vi "DevicesManager.vi"(8 "error in (no error)":errorcluster, 10 "Notifiers":T2, 11 "All Message Queue Cluster":T3) -> (0 "error out":errorcluster)   [LabVIEW 2013]
doc: "Ce VI a pour but de géré la connection des différents appareils.\n- Il permet de les connecté en fonction de leur port.\n- Il indique s'il se sont bien connecter et si tout se passe bien."
uses:
  Lib QMH/AllMessageQueue Cluster.ctl
  Lib QMH/Message Cluster.ctl
  Lib Notifier/Notifier.ctl
  Manager UI Data.ctl
  Lib QMH/MessageQueues.lvlib
  Lib Notifier/Notifier.lvlib
panel:
  in  "Port Number Slit":T1(ring)=enum."COM3"
  out "Camera Initialized":bool
  out "Laser Initialized":bool
  out "Status Camera":string
  out "Status Laser":string
  in  "Connect Laser":bool
  in  "Connect Camera":bool
  # "Camera"
  # "Laser"
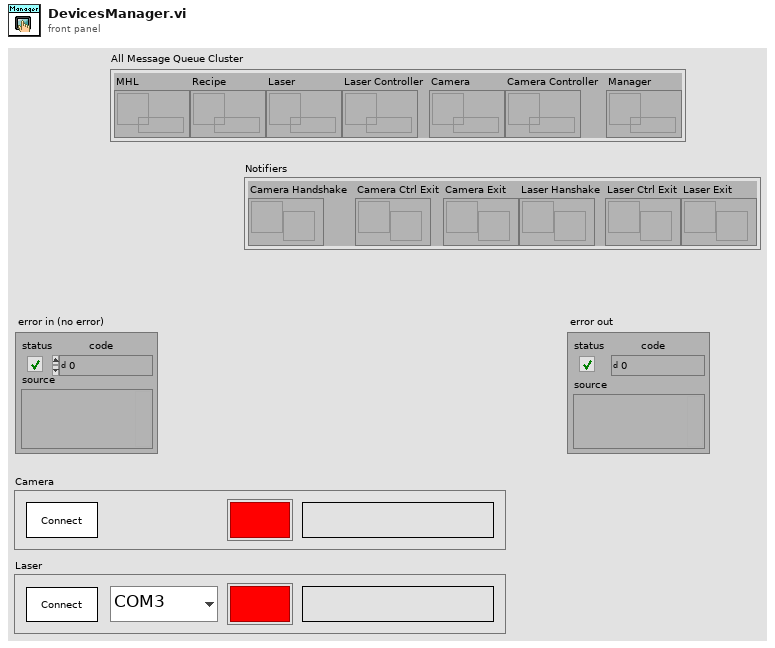
[diagram p1: front panel]
types:
  T1 = enum16{"COM1", "COM2", "COM3", "COM4", "COM5", "COM6", "COM7", "COM8", "COM9", "COM10", "COM11", "COM12", "COM13", "COM14", "COM15", "COM16", "COM17", "COM18", "COM19", "COM20", "COM21", "COM22", "COM23", "COM24", "COM25", "COM26", "COM27", "COM28", "COM29", "COM30"}
  T2 = typedef "Notifier.lvlib/Notifier.ctl" = cluster{"Camera Handshake":refnum<notifier>, "Camera Ctrl Exit":refnum<notifier>, "Camera Exit":refnum<notifier>, "Laser Hanshake":refnum<notifier>, "Laser Ctrl Exit":refnum<notifier>, "Laser Exit":refnum<notifier>}
  T3 = typedef "MessageQueues.lvlib/AllMessageQueue Cluster.ctl" = cluster{"MHL":refnum<queue>, "Recipe":refnum<queue>, "Laser":refnum<queue>, "Laser Controller":refnum<queue>, "Camera":refnum<queue>, "Camera Controller":refnum<queue>, "Manager":refnum<queue>}
  T4 = typedef "Manager UI Data.ctl" = cluster{"Camera Initialized":bool, "Status Camera":string, "Laser Initialized":bool, "Status Laser":string}
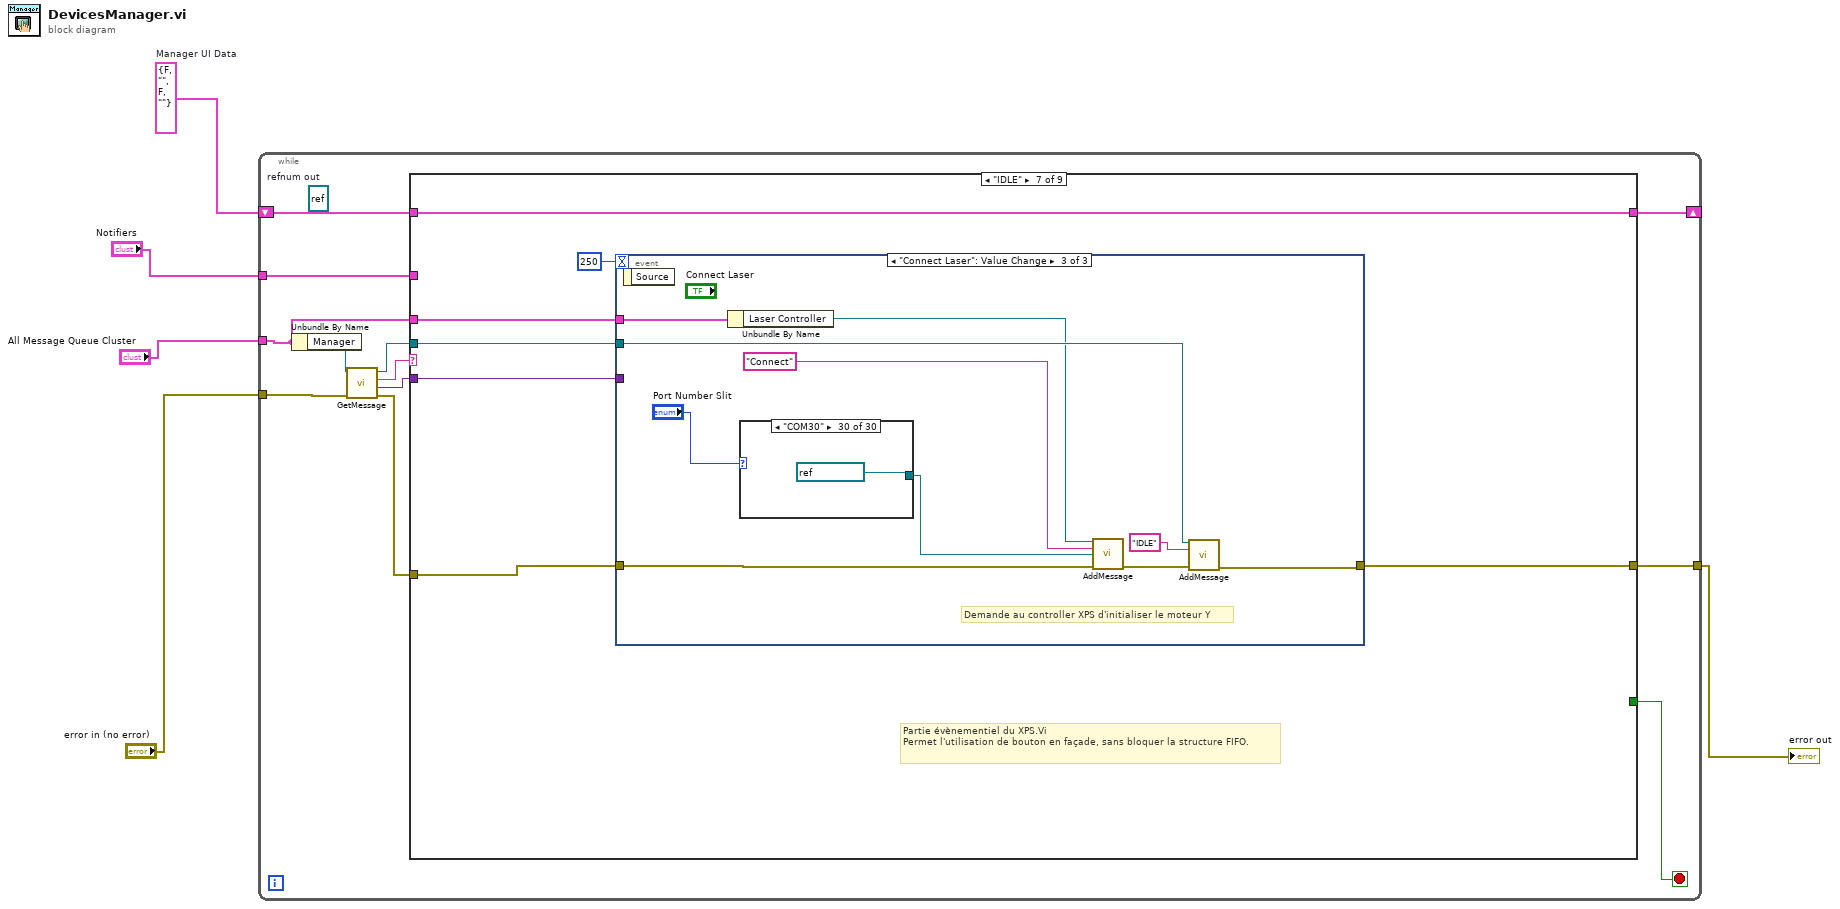
[diagram p0: block diagram]
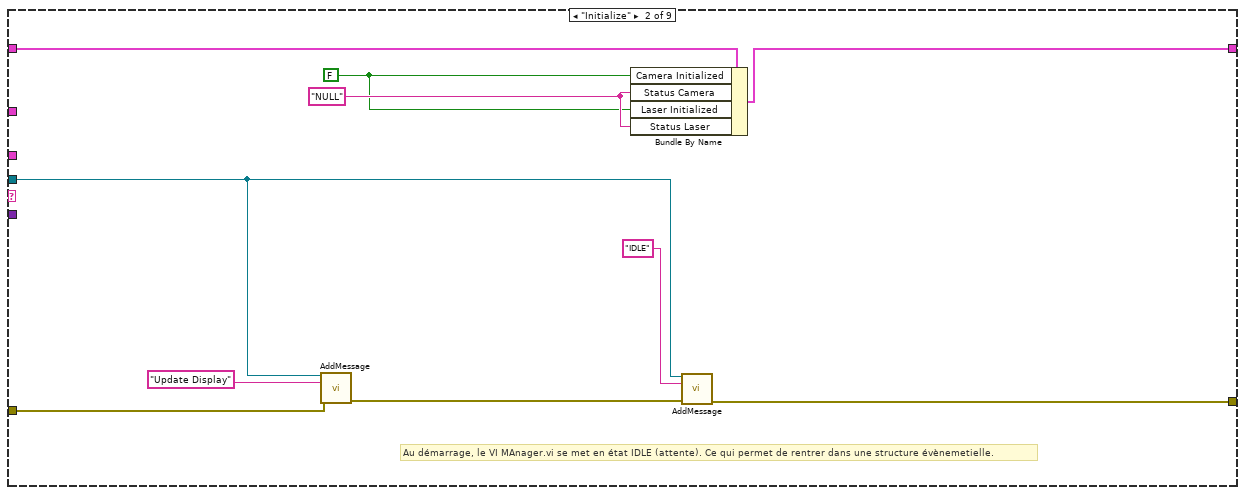
[diagram p3: hidden frame]
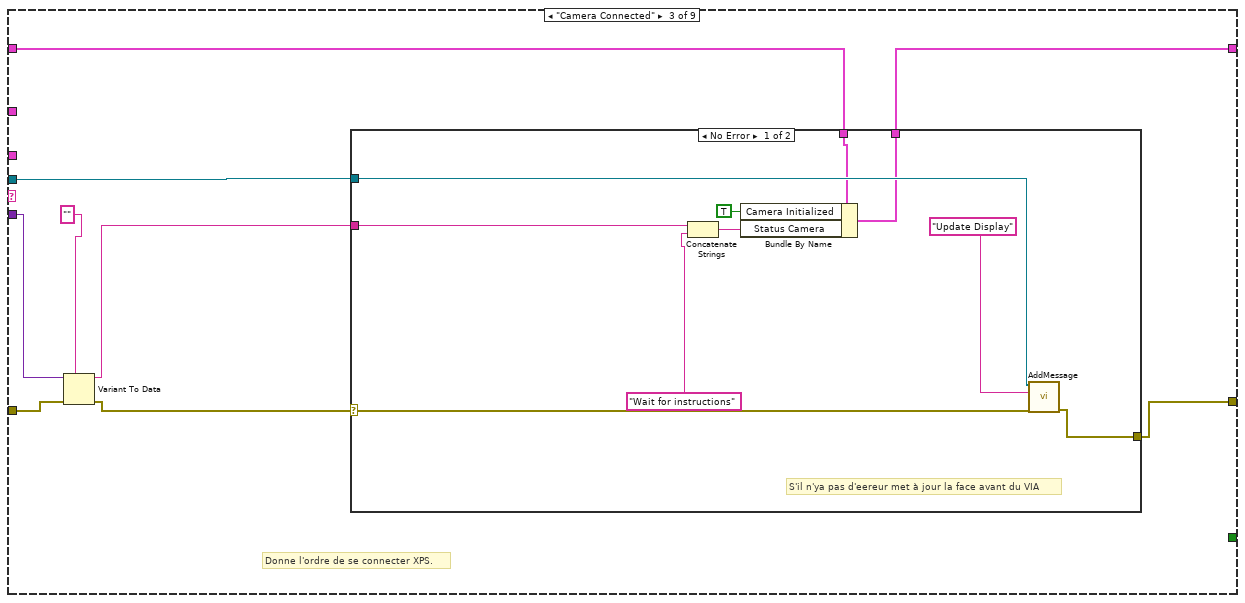
[diagram p4: hidden frame]
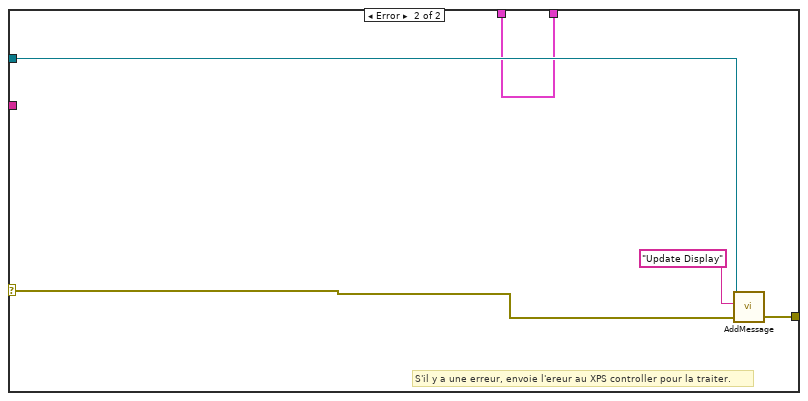
[diagram p5: hidden frame]
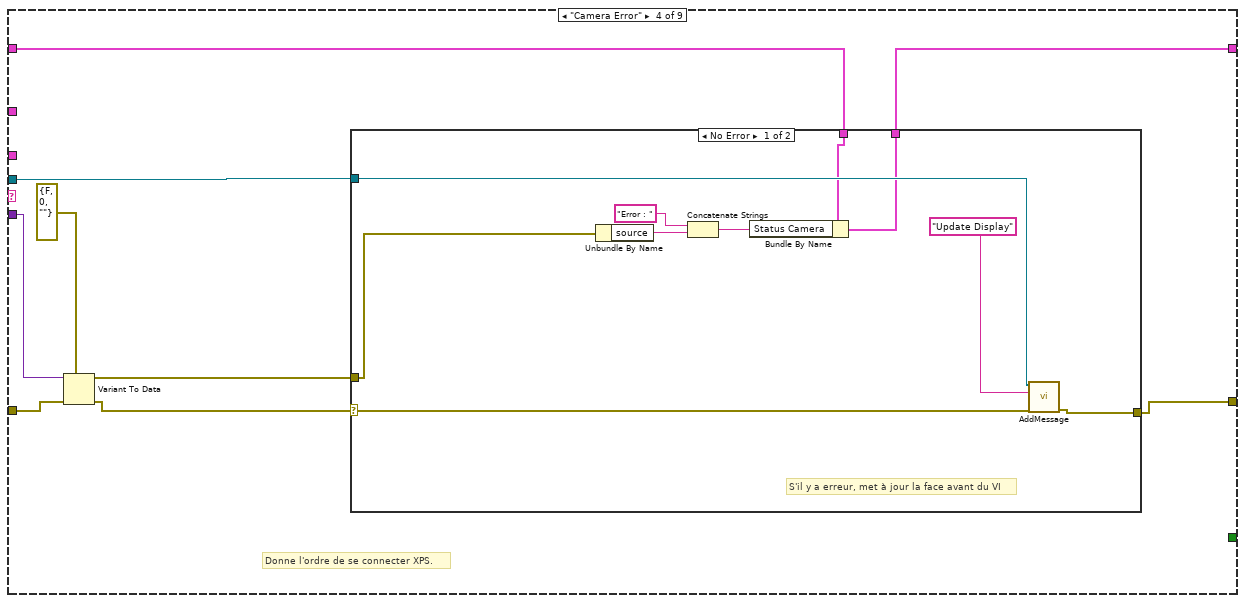
[diagram p6: hidden frame]
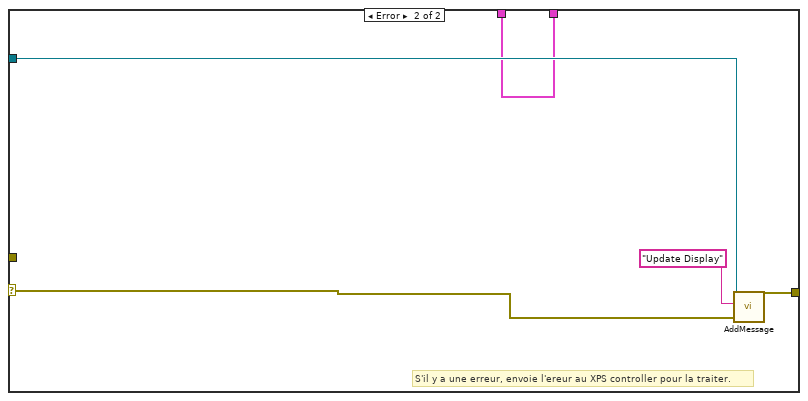
[diagram p7: hidden frame]
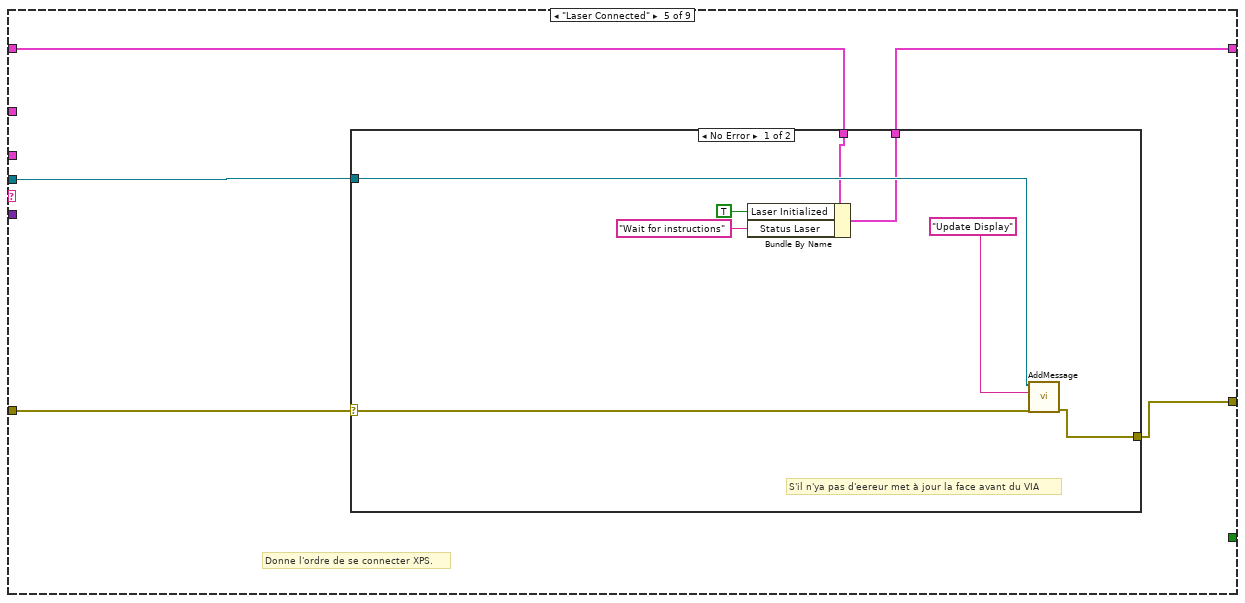
[diagram p8: hidden frame]
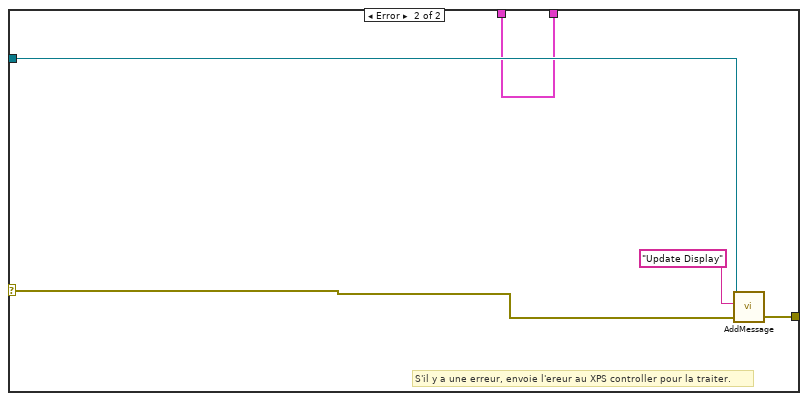
[diagram p9: hidden frame]
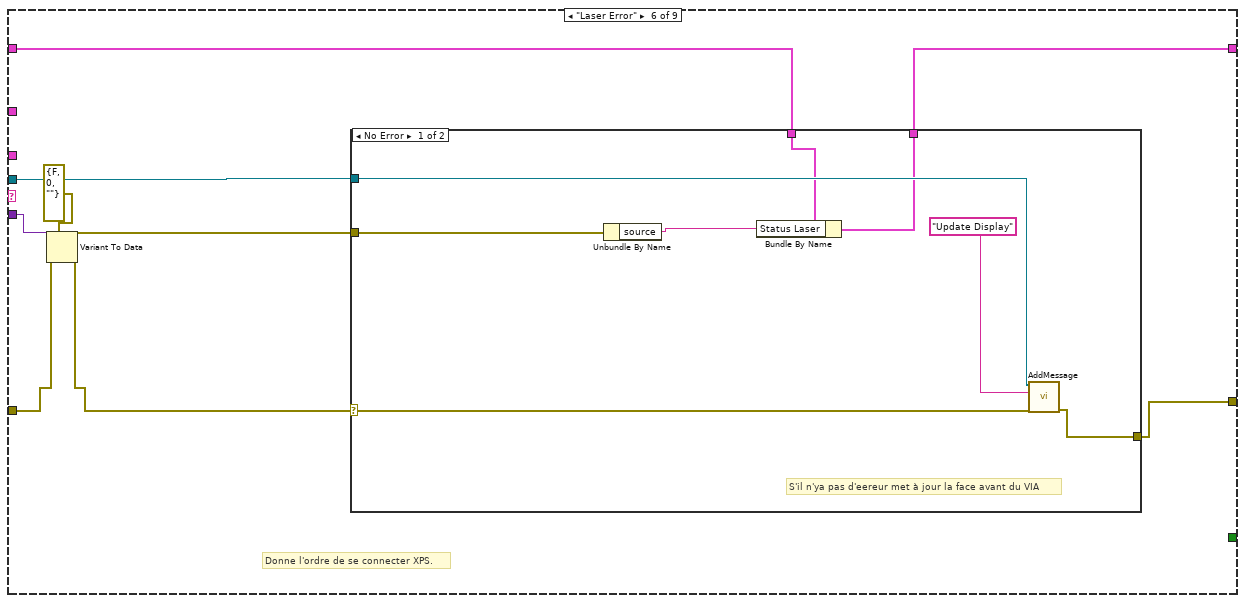
[diagram p10: hidden frame]
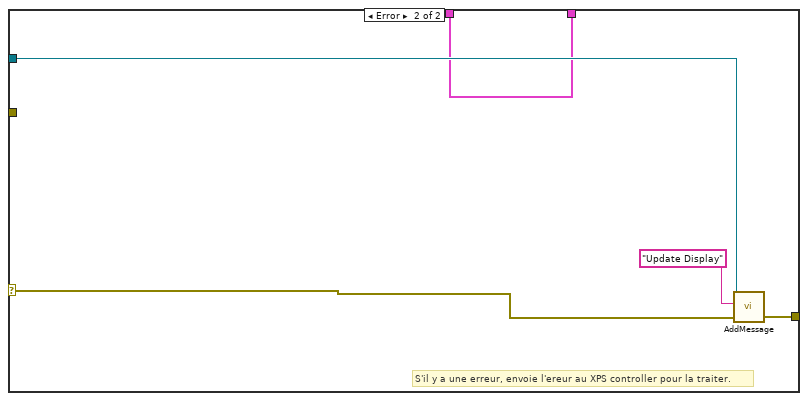
[diagram p11: hidden frame]
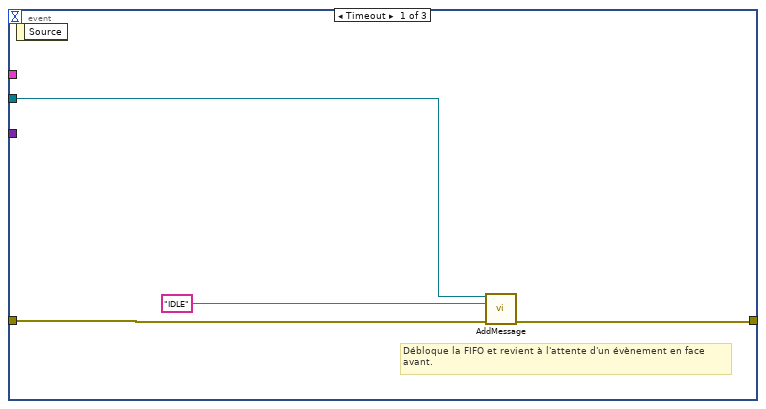
[diagram p12: hidden frame]
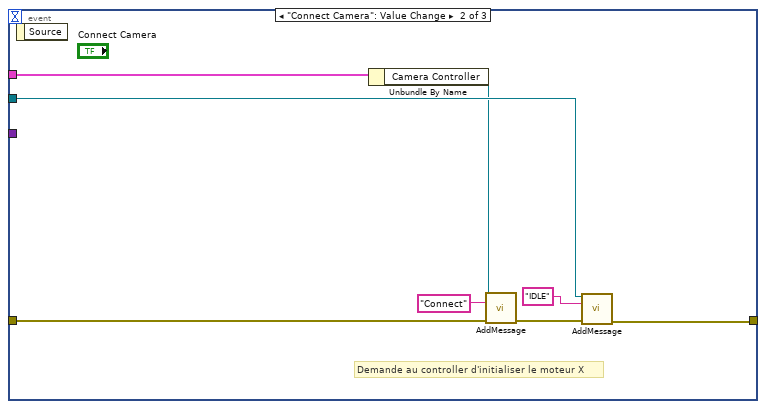
[diagram p13: hidden frame]
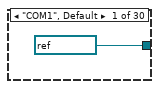
[diagram p14: hidden frame]
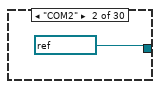
[diagram p15: hidden frame]
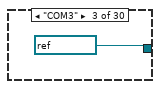
[diagram p16: hidden frame]
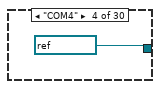
[diagram p17: hidden frame]
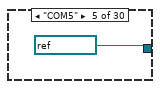
[diagram p18: hidden frame]
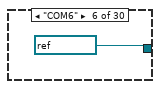
[diagram p19: hidden frame]
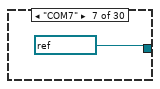
[diagram p20: hidden frame]
diagram:
  w1 = T4 {"Camera Initialized"=FALSE, "Status Camera"="", "Laser Initialized"=FALSE, "Status Laser"=""}  # Manager UI Data
  (unwired) refnum<file> refnum  # refnum out
  n1 = while {
    tunnel: "All Message Queue Cluster" -> [w6]
    tunnel: "Notifiers" -> [w17]
    tunnel: "error in (no error)" -> [w11]
    tunnel: [w10] -> w2
    shift-right: [w7] -> _
    shift-left: w1 -> [w8]
    stop <- w9 stop-if-true
    n2 = Unbundle By Name(w6) -> ("Manager"=w16:refnum<queue>)
    n3 = call "GetMessage.vi"("entrée d'erreur"=w11, "Message queue"=w16) -> ("sortie d'erreur"=w12:errorcluster, "Data"=w13:variant, "Message"=w14:string, "Dup Message Queue"=w15:refnum<queue>)  [unwired: 6 in]
    n4 = case shown="\"IDLE\"" w14 {
      tunnel: w17 -> [_ _ _ _ _ _ _ _ _]
      tunnel: w15 -> [_ w21 w38 w62 w82 w104 w123 _ w185]
      tunnel: w13 -> [_ _ w32 w56 _ w98 w122 _ _]
      tunnel: w12 -> [w19 w23 w34 w58 w78 w100 w121 w182 w186]
      tunnel: [w19 w28 w37 w61 w81 w103 w120 w182 w183] -> w10
      tunnel: [_ _ _ _ _ _ _ _ TRUE] -> w9
      tunnel: w8 -> [w18 w27 w36 w60 w80 w102 w119 w181 w184]
      tunnel: [w18 w26 w35 w59 w79 w101 w119 w181 w184] -> w7
      tunnel: w6 -> [_ _ _ _ _ _ w118 _ _]
      frame Default {
        # "ne fait rien si le message dépilé n'existe pas"
      }
      frame "Initialize" {
        w25 = "NULL" ("Status Spectro")
        w24 = FALSE ("Spectro Initialized")
        # "Au démarrage, le VI MAnager.vi se met en état IDLE (attente). Ce qui permet de rentrer dans une structure évènemetielle."
        n5 = call "AddMessage.vi"("Message queue"=w21, "Message"="Update Display", "entrée d'erreur (pas d'erreur)"=w23) -> ("error out"=w22:errorcluster)  [unwired: 11 in, 1 out]
        n6 = Bundle By Name(cluster=w27, "Camera Initialized"=w24, "Status Camera"=w25, "Laser Initialized"=w24, "Status Laser"=w25) -> (w26:T4)
        n7 = call "AddMessage.vi"("Message queue"=w21, "Message"="IDLE", "entrée d'erreur (pas d'erreur)"=w22) -> ("error out"=w28:errorcluster)  [unwired: 11 in, 1 out]
      }
      frame "Camera Connected" {
        # "Donne l'ordre de se connecter XPS."
        n8 = Variant To Data(error in=w34, type="", Variant=w32) -> (data=w30:string, error out=w33:errorcluster)
        n9 = case shown="No Error" w33 {
          selector: w33 -> [w46 w49]
          tunnel: w38 -> [w48 w53]
          tunnel: [w45 w51] -> w37
          tunnel: w36 -> [w44 w50]
          tunnel: [w43 w50] -> w35
          tunnel: w30 -> [w39 _]
          frame No Error {
            # "S'il n'ya pas d'eereur met à jour la face avant du VIA"
            n10 = Concatenate Strings(w39, "Wait for instructions" ("Status Spectro")) -> (w40:string)
            n11 = Bundle By Name(cluster=w44, "Camera Initialized"=TRUE ("Spectro Initialized"), "Status Camera"=w40) -> (w43:T4)
            n12 = call "AddMessage.vi"("Message queue"=w48, "Message"="Update Display", "entrée d'erreur (pas d'erreur)"=w46) -> ("error out"=w45:errorcluster)  [unwired: 11 in, 1 out]
          }
          frame Error {
            # "S'il y a une erreur, envoie l'ereur au XPS controller pour la traiter."
            n13 = call "AddMessage.vi"("Message queue"=w53, "Message"="Update Display", "entrée d'erreur (pas d'erreur)"=w49) -> ("error out"=w51:errorcluster)  [unwired: 11 in, 1 out]
          }
        }
      }
      frame "Camera Error" {
        # "Donne l'ordre de se connecter XPS."
        n14 = Variant To Data(error in=w58, type=errorcluster {"status"=FALSE, "code"=0, "source"=""} ("error out"), Variant=w56) -> (data=w54:errorcluster, error out=w57:errorcluster)
        n15 = case shown="No Error" w57 {
          selector: w57 -> [w70 w73]
          tunnel: w62 -> [w72 w77]
          tunnel: [w69 w75] -> w61
          tunnel: w60 -> [w68 w74]
          tunnel: [w67 w74] -> w59
          tunnel: w54 -> [w65 _]
          frame No Error {
            # "S'il y a erreur, met à jour la face avant du VI"
            n16 = Unbundle By Name(w65) -> ("source"=w64:string)
            n17 = Concatenate Strings("Error : " ("string"), w64) -> (w66:string)
            n18 = Bundle By Name(cluster=w68, "Status Camera"=w66) -> (w67:T4)
            n19 = call "AddMessage.vi"("Message queue"=w72, "Message"="Update Display", "entrée d'erreur (pas d'erreur)"=w70) -> ("error out"=w69:errorcluster)  [unwired: 11 in, 1 out]
          }
          frame Error {
            # "S'il y a une erreur, envoie l'ereur au XPS controller pour la traiter."
            n20 = call "AddMessage.vi"("Message queue"=w77, "Message"="Update Display", "entrée d'erreur (pas d'erreur)"=w73) -> ("error out"=w75:errorcluster)  [unwired: 11 in, 1 out]
          }
        }
      }
      frame "Laser Connected" {
        # "Donne l'ordre de se connecter XPS."
        n21 = case shown="No Error" w78 {
          selector: w78 -> [w88 w91]
          tunnel: w82 -> [w90 w95]
          tunnel: [w87 w93] -> w81
          tunnel: w80 -> [w86 w92]
          tunnel: [w85 w92] -> w79
          frame No Error {
            # "S'il n'ya pas d'eereur met à jour la face avant du VIA"
            n22 = Bundle By Name(cluster=w86, "Laser Initialized"=TRUE ("Spectro Initialized"), "Status Laser"="Wait for instructions" ("Status Spectro")) -> (w85:T4)
            n23 = call "AddMessage.vi"("Message queue"=w90, "Message"="Update Display", "entrée d'erreur (pas d'erreur)"=w88) -> ("error out"=w87:errorcluster)  [unwired: 11 in, 1 out]
          }
          frame Error {
            # "S'il y a une erreur, envoie l'ereur au XPS controller pour la traiter."
            n24 = call "AddMessage.vi"("Message queue"=w95, "Message"="Update Display", "entrée d'erreur (pas d'erreur)"=w91) -> ("error out"=w93:errorcluster)  [unwired: 11 in, 1 out]
          }
        }
      }
      frame "Laser Error" {
        # "Donne l'ordre de se connecter XPS."
        n25 = Variant To Data(error in=w100, type=errorcluster {"status"=FALSE, "code"=0, "source"=""} ("error out"), Variant=w98) -> (data=w96:errorcluster, error out=w99:errorcluster)
        n26 = case shown="No Error" w99 {
          selector: w99 -> [w110 w113]
          tunnel: w104 -> [w112 w117]
          tunnel: [w109 w115] -> w103
          tunnel: w102 -> [w108 w114]
          tunnel: [w107 w114] -> w101
          tunnel: w96 -> [w106 _]
          frame No Error {
            # "S'il n'ya pas d'eereur met à jour la face avant du VIA"
            n27 = Unbundle By Name(w106) -> ("source"=w105:string)
            n28 = Bundle By Name(cluster=w108, "Status Laser"=w105) -> (w107:T4)
            n29 = call "AddMessage.vi"("Message queue"=w112, "Message"="Update Display", "entrée d'erreur (pas d'erreur)"=w110) -> ("error out"=w109:errorcluster)  [unwired: 11 in, 1 out]
          }
          frame Error {
            # "S'il y a une erreur, envoie l'ereur au XPS controller pour la traiter."
            n30 = call "AddMessage.vi"("Message queue"=w117, "Message"="Update Display", "entrée d'erreur (pas d'erreur)"=w113) -> ("error out"=w115:errorcluster)  [unwired: 11 in, 1 out]
          }
        }
      }
      frame "IDLE" {
        # "Partie évènementiel du XPS.Vi\nPermet l'utilisation de bouton en façade, sans bloquer la structure FIFO."
        n31 = event shown="[2] \"Connect Laser\": Value Change" {
          selector: _ -> [_ _ _]
          dyn-events: _ -> [_ _ _]
          timeout: 250 -> [_ _ _]
          tunnel: w123 -> [w128 w131 w141]
          tunnel: w122 -> [_ _ _]
          tunnel: w121 -> [w127 w136 w146]
          tunnel: [w126 w133 w143] -> w120
          tunnel: w118 -> [_ w130 w140]
          event Timeout {
            # "Débloque la FIFO et revient à l'attente d'un évènement en face\navant."
            n32 = event-data() -> ()  [unwired: 1 in, 1 out]
            n33 = call "AddMessage.vi"("Message queue"=w128, "Message"="IDLE", "entrée d'erreur (pas d'erreur)"=w127) -> ("error out"=w126:errorcluster)  [unwired: 11 in, 1 out]
          }
          event "Connect Camera": Value Change {
            # "Demande au controller d'initialiser le moteur X"
            n34 = event-data() -> ()  [unwired: 1 in, 1 out]
            n35 = Unbundle By Name(w130) -> ("Camera Controller"=w129:refnum<queue>)
            n36 = call "AddMessage.vi"("Message queue"=w129, "Message"="Connect", "entrée d'erreur (pas d'erreur)"=w136) -> ("error out"=w134:errorcluster)  [unwired: 11 in, 1 out]
            n37 = call "AddMessage.vi"("Message queue"=w131, "Message"="IDLE", "entrée d'erreur (pas d'erreur)"=w134) -> ("error out"=w133:errorcluster)  [unwired: 11 in, 1 out]
          }
          event "Connect Laser": Value Change {
            # "Demande au controller XPS d'initialiser le moteur Y"
            n38 = event-data() -> ()  [unwired: 1 in, 1 out]
            n39 = Unbundle By Name(w140) -> ("Laser Controller"=w139:refnum<queue>)
            n40 = case shown="\"COM30\"" "Port Number Slit" {
              tunnel: [refnum<visa-resource-name> "COM1" ("VISA resource name out") refnum<visa-resource-name> "COM2" ("VISA resource name out") refnum<visa-resource-name> "COM3" ("VISA resource name out") refnum<visa-resource-name> "COM4" ("VISA resource name out") refnum<visa-resource-name> "COM5" ("VISA resource name out") refnum<visa-resource-name> "COM6" ("VISA resource name out") refnum<visa-resource-name> "COM7" ("VISA resource name out") refnum<visa-resource-name> "COM8" ("VISA resource name out") refnum<visa-resource-name> "COM9" ("VISA resource name out") refnum<visa-resource-name> "COM10" ("VISA resource name out") refnum<visa-resource-name> "COM11" ("VISA resource name out") refnum<visa-resource-name> "COM12" ("VISA resource name out") refnum<visa-resource-name> "COM13" ("VISA resource name out") refnum<visa-resource-name> "COM14" ("VISA resource name out") refnum<visa-resource-name> "COM15" ("VISA resource name out") refnum<visa-resource-name> "COM16" ("VISA resource name out") refnum<visa-resource-name> "COM17" ("VISA resource name out") refnum<visa-resource-name> "COM18" ("VISA resource name out") refnum<visa-resource-name> "COM19" ("VISA resource name out") refnum<visa-resource-name> "COM20" ("VISA resource name out") refnum<visa-resource-name> "COM21" ("VISA resource name out") refnum<visa-resource-name> "COM22" ("VISA resource name out") refnum<visa-resource-name> "COM23" ("VISA resource name out") refnum<visa-resource-name> "COM24" ("VISA resource name out") refnum<visa-resource-name> "COM25" ("VISA resource name out") refnum<visa-resource-name> "COM26" ("VISA resource name out") refnum<visa-resource-name> "COM27" ("VISA resource name out") refnum<visa-resource-name> "COM28" ("VISA resource name out") refnum<visa-resource-name> "COM29" ("VISA resource name out") refnum<visa-resource-name> "COM30" ("VISA resource name out")] -> w137
              frame "COM1", Default {
              }
              frame "COM2" {
              }
              frame "COM3" {
              }
              frame "COM4" {
              }
              frame "COM5" {
              }
              frame "COM6" {
              }
              frame "COM7" {
              }
              frame "COM8" {
              }
              frame "COM9" {
              }
              frame "COM10" {
              }
              frame "COM11" {
              }
              frame "COM12" {
              }
              frame "COM13" {
              }
              frame "COM14" {
              }
              frame "COM15" {
              }
              frame "COM16" {
              }
              frame "COM17" {
              }
              frame "COM18" {
              }
              frame "COM19" {
              }
              frame "COM20" {
              }
              frame "COM21" {
              }
              frame "COM22" {
              }
              frame "COM23" {
              }
              frame "COM24" {
              }
              frame "COM25" {
              }
              frame "COM26" {
              }
              frame "COM27" {
              }
              frame "COM28" {
              }
              frame "COM29" {
              }
              frame "COM30" {
              }
            }
            n41 = call "AddMessage.vi"("Message queue"=w139, "Message"="Connect", "Data"=w137, "entrée d'erreur (pas d'erreur)"=w146) -> ("error out"=w144:errorcluster)  [unwired: 10 in, 1 out]
            n42 = call "AddMessage.vi"("Message queue"=w141, "Message"="IDLE", "entrée d'erreur (pas d'erreur)"=w144) -> ("error out"=w143:errorcluster)  [unwired: 11 in, 1 out]
          }
        }
      }
      frame "Update Display" {
        # "Met à jour les valeur de status"
        n43 = Unbundle By Name(w181) -> ("Camera Initialized"=→"Camera Initialized":bool, "Status Camera"=→"Status Camera":string, "Laser Initialized"=→"Laser Initialized":bool, "Status Laser"=→"Status Laser":string)
      }
      frame "Exit" {
        n44 = Release Queue(queue=w185, error in (no error)=w186) -> (error out=w183:errorcluster)  [unwired: 1 in, 2 out]
      }
    }
  }
  "error out" <- w2
